vi "Renishaw-XL80_Reinitialize.vi"(8 "error in (no error)":errorcluster, 11 "Renishaw-XL80_EMU in":refnum<class "Renishaw-XL80_EMU.lvclass">) -> (0 "error out":errorcluster, 3 "Renishaw-XL80_EMU out":refnum<class "Renishaw-XL80_EMU.lvclass">)   [LabVIEW 2024, in "Renishaw-XL80_EMU.lvclass"]
uses:
  Renishaw-XL80_EMU.lvclass
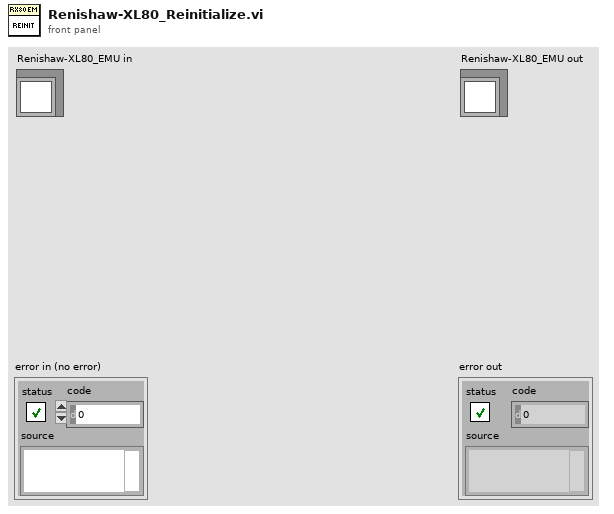
[diagram p1: front panel]
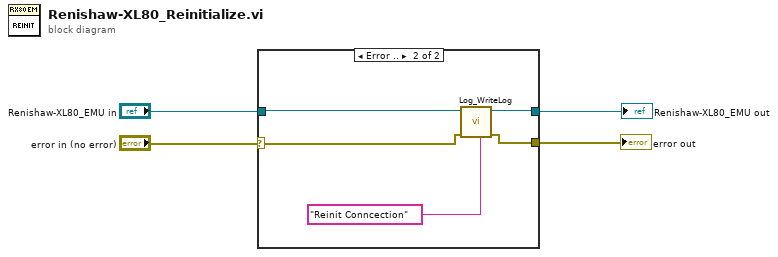
[diagram p0: block diagram]
diagram:
  n1 = case shown="Error .." "error in (no error)" {
    selector: "error in (no error)" -> [w5 w9]
    tunnel: [w6 w8] -> w4
    tunnel: "Renishaw-XL80_EMU in" -> [w6 w10]
    tunnel: [w5 w7] -> w1
    frame No Error {
    }
    frame Error {
      n2 = call-dynamic "Log_WriteLog.vi"("Additional text"="Reinit Conncection", "error in (no error)"=w9, "Log in"=w10) -> ("error out"=w7:errorcluster, "Log out"=w8:refnum<class "Renishaw-XL80_EMU.lvclass">)  [unwired: 7 in]
    }
  }
  "error out" <- w1
  "Renishaw-XL80_EMU out" <- w4
